vi "TIO Stream Open.vi"(7 "Port timeout":u32=500, 10 "Default baud":u32=115200, 11 "URL":refnum<visa-resource-name>="tcp://localhost") -> (0 "error out":errorcluster, 1 "Connected":bool=TRUE, 3 "TS Connection":T1={"Type"=enum."TCP", "Serial"="serial:///dev/cu.usbserial-00000", "TCP"=refnum, "Timeout"=500})   [LabVIEW 2017]
uses:
  <vilib>/Instr/_visa.llb/VISA Configure Serial Port (Instr).vi
  <instrlib>/tio-labview/TIO Library/Socket/Helpers/TIO Serial Port Discovery.vi
panel:
  in  "Default Port":i32=7855
  in  "error in (no error)":errorcluster
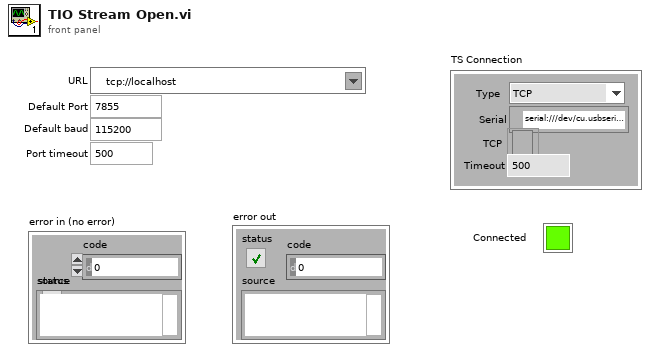
[diagram p1: front panel]
types:
  T1 = cluster{"Type":enum16{"TCP", "Serial"}, "Serial":refnum<visa-resource-name>, "TCP":refnum<k5>, "Timeout":u32}
  T2 = cluster{"Type":u16, "VISA resource name out":refnum<visa-resource-name>, "connection ID":refnum<k5>, "Port timeout":u32}
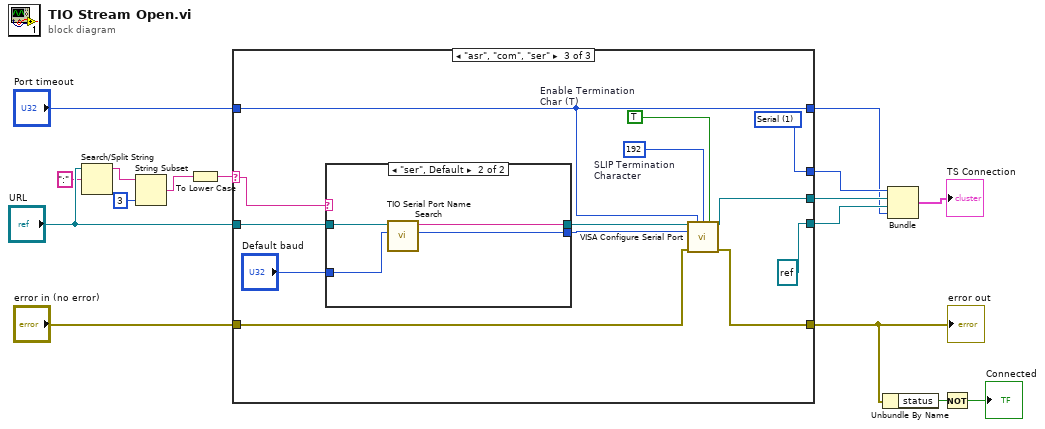
[diagram p0: block diagram]
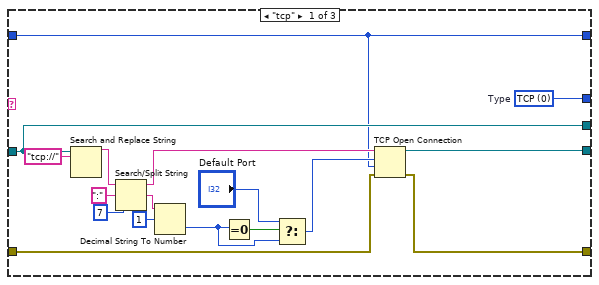
[diagram p2: hidden frame]
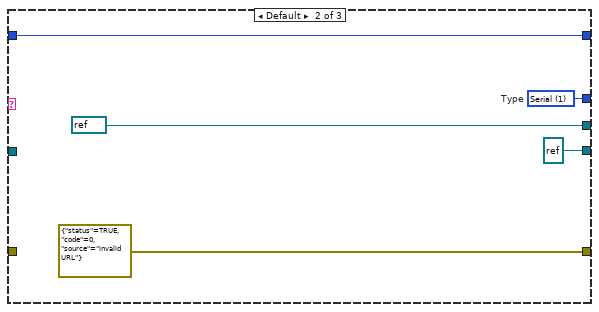
[diagram p3: hidden frame]
diagram:
  n1 = Search/Split String(string="URL", search string/char (-)=":") -> (substring before match=w14:string)  [unwired: 1 in, 2 out]
  n2 = String Subset(string=w14, length (rest)=3 ("length (rest)")) -> (substring=w11:string)  [unwired: 1 in]
  n3 = To Lower Case(string=w11) -> (all lower case string=w12:string)
  n4 = case shown="\"asr\", \"com\", \"ser\"" w12 {
    selector: w12 -> [_ _ w46]
    tunnel: [w22 errorcluster {"status"=TRUE, "code"=0, "source"="invalid URL"} ("error out") w45] -> w10
    tunnel: [w20 refnum<visa-resource-name> refnum ("VISA resource name out") w44] -> w5
    tunnel: "URL" -> [w20 _ w49]
    tunnel: "error in (no error)" -> [w23 _ w43]
    tunnel: [w21 refnum<k5> refnum ("connection ID") refnum<k5> refnum ("connection ID")] -> w4
    tunnel: [w19 w36 w41] -> w7
    tunnel: "Port timeout" -> [w17 w34 w39]
    tunnel: [w17 w34 w39] -> w1
    frame "tcp" {
      w19 = u16 0 items=["TCP", "Serial"]  # Type
      n5 = Search and Replace String(input string=w20, search string="tcp://") -> (result string=w30:string)  [unwired: 6 in, 3 out]
      n6 = Search/Split String(string=w30, search string/char (-)=":", offset (0)=7) -> (substring before match=w24:string, match + rest of string=w29:string)  [unwired: 1 out]
      n7 = Decimal String To Number(string=w29, offset=1) -> (number=w27:i32)  [unwired: 1 in, 1 out]
      n8 = Equal To 0?(x=w27) -> (x = 0?=w26:bool)
      n9 = Select(t="Default Port", s=w26, f=w27) -> (s? t:f=w18:i32)
      n10 = TCP Open Connection(address=w24, remote port or service name=w18, timeout ms (60000)=w17, error in (no error)=w23) -> (connection ID=w21:refnum<k5>, error out=w22:errorcluster)  [unwired: 1 in]
    }
    frame Default {
      w36 = u16 1 items=["TCP", "Serial"]  # Type
    }
    frame "asr", "com", "ser" {
      w41 = u16 1 items=["TCP", "Serial"] ("Type")
      w50 = TRUE  # Enable Termination Char (T)
      w51 = u8 192  # SLIP Termination Character
      n11 = case shown="\"ser\", Default" w46 {
        tunnel: w49 -> [w53 w57]
        tunnel: [w53 w56] -> w48
        tunnel: [w52 w55] -> w47
        tunnel: "Default baud" -> [w52 w54]
        frame "asr", "com" {
        }
        frame "ser", Default {
          n12 = call <instrlib>:"TIO Serial Port Name Search.vi"("Default baud"=w54, "String"=w57) -> ("Baud"=w55:i32, "VISA Resource"=w56:string)  [unwired: 7 in, 1 out]
        }
      }
      n13 = call-poly "VISA Configure Serial Port"("VISA resource name"=w48, "timeout (10sec)"=w39, "termination char\n(0xA = '\\n' = LF)"=w51, "Enable Termination\nChar (T)"=w50, "baud rate (9600)"=w47, "error in (no error)"=w43) -> ("VISA resource name out"=w44:refnum<visa-resource-name>, "error out"=w45:errorcluster)  [unwired: 8 in]
    }
  }
  "error out" <- w10
  n14 = Unbundle By Name(w10) -> ("status"=w9:bool)
  n15 = Bundle("Type"=w7, "VISA resource name out"=w5, "connection ID"=w4, "Port timeout"=w1) -> (→"TS Connection":T2)  [unwired: 1 in]
  n16 = Not(x=w9) -> (.not. x?=→"Connected":bool)
